vi "Channel Selection Dialog.vi"(7 "DisplayFilter":u8(ring)=7 items=["K_CHAN_R", "K_CHAN_W", "K_CHAN_RW", "K_CHAN_VOLT", "K_CHAN_FAULT", "K_ALL", "K_CUSTOM", "K_CHAN_R_VIS", "K_CHAN_W_VIS", "K_CHAN_RW_VIS", "K_CHAN_VOLT_VIS", "K_CHAN_FAULT_VIS"], 8 "error in (no error)":errorcluster, 9 "NIVS.System Definition Root":refnum<k24>, 10 "Start NodePath":string, 11 "Start NodePathArray":string[](array[string])) -> (0 "error out":errorcluster, 1 "Cancelled?":bool, 2 "Selected NodePath":string, 3 "Selected NodePathArray":string[](array[string]))   [LabVIEW 2011]
doc: "Use this template to create a dialog box with event handling."
uses:
  NationalInstruments.VeriStand.SystemStorageUI
  NationalInstruments.VeriStand.SystemStorage
  <vilib>/NI Veristand/UI Controls/Single Node Browser/NI_VS UI Single Node Browser.lvlib
panel:
  in  "Cancel":bool
  in  "Ok":bool
  in  "Selected Channel":refnum<k24>(container)
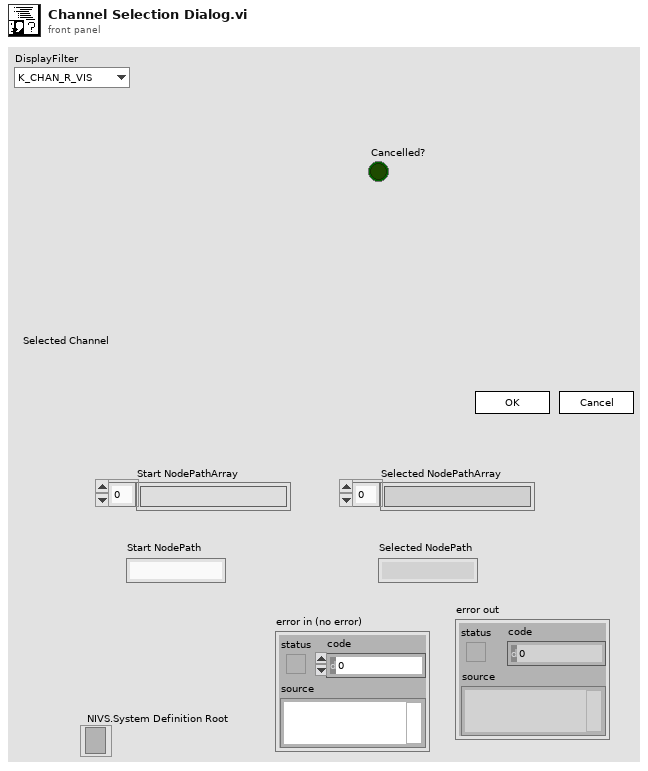
[diagram p1: front panel]
types:
  T1 = typedef "NI_VS UI Single Node Browser.lvlib/Callback Type.ctl" = cluster{"Net Callbacks":refnum<k27>[], "Event":refnum<user-event>}
  T2 = typedef "NI_VS UI Single Node Browser.lvlib/Node Ref.ctl" = refnum<k24>
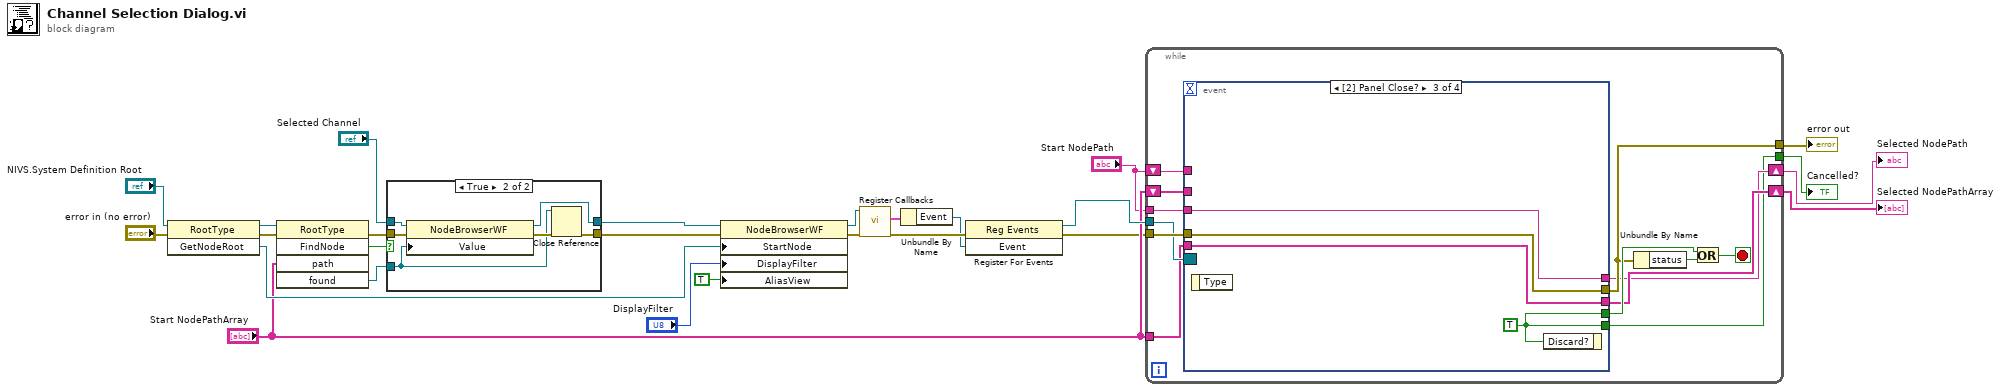
[diagram p0: block diagram]
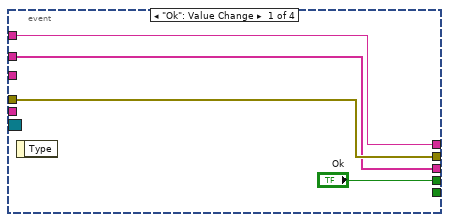
[diagram p3: hidden frame]
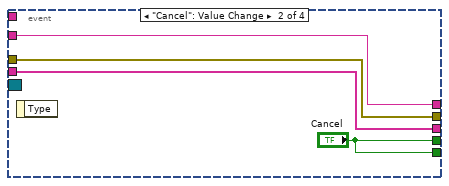
[diagram p4: hidden frame]
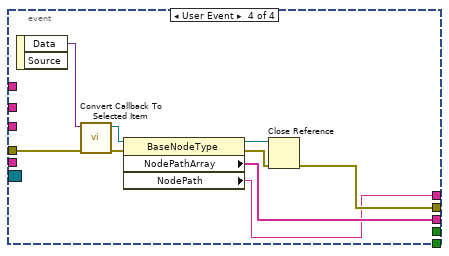
[diagram p5: hidden frame]
diagram:
  n1 = invoke class="RootType" method="GetNodeRoot"(reference="NIVS.System Definition Root", error in="error in (no error)") -> (reference out=w20:refnum<k24>, error out=w21:errorcluster, "GetNodeRoot"=w19:refnum<k24>)  [unwired: 1 in]
  n2 = invoke class="RootType" method="FindNode"(reference=w20, error in=w21, "path"="Start NodePathArray") -> (error out=w12:errorcluster, "FindNode"=w10:bool, "found"=w13:refnum<k24>)  [unwired: 2 in, 2 out]
  n3 = case shown="True" w10 {
    tunnel: w13 -> [_ w29]
    tunnel: w12 -> [w28 w30]
    tunnel: [w28 w33] -> w11
    tunnel: "Selected Channel" -> [w27 w32]
    tunnel: [w27 w31] -> w9
    frame False {
    }
    frame True {
      n4 = property class="NodeBrowserWF"(reference=w32, error in=w30, "Value"=w29) -> (reference out=w31:refnum<k24>, error out=w34:errorcluster)
      n5 = Close Reference(reference=w29, error in (no error)=w34) -> (error out=w33:errorcluster)
    }
  }
  n6 = property class="NodeBrowserWF"(reference=w9, error in=w11, "StartNode"=w19, "DisplayFilter"="DisplayFilter", "AliasView"=TRUE) -> (reference out=w16:refnum<k24>, error out=w17:errorcluster)
  n7 = call <vilib>:"Register Callbacks.vi"("error in (no error)"=w17, "Single Node Browser"=w16) -> ("error out"=w25:errorcluster, "Callbacks"=w18:T1)  [unwired: 7 in, 1 out]
  n8 = Unbundle By Name(w18) -> ("Event"=w8:refnum<user-event>)
  n9 = register-events(error in=w25, w8) -> (reference out=w24:refnum<event-registration>, error out=w1:errorcluster)  [unwired: 1 in]
  n10 = while {
    tunnel: [w45] -> w26
    tunnel: w1 -> [w46]
    tunnel: w24 -> [w42]
    shift-right: [w41] -> w7
    shift-left: "Start NodePathArray" -> [w40]
    tunnel: "Start NodePathArray" -> [w39]
    shift-right: [w38] -> w5
    shift-left: "Start NodePath" -> [w37]
    tunnel: "Start NodePath" -> [w36]
    tunnel: [w35] -> w3
    stop <- w44 stop-if-true
    n11 = event shown="[2] Panel Close?" {
      selector: w42 -> [_ _ _ _]
      dyn-events: _ -> [_ _ _ _]
      timeout: _ -> [_ _ _ _]
      tunnel: ["Ok" "Cancel" w56 _] -> w47
      tunnel: [w51 w55 w59 w66] -> w45
      tunnel: w46 -> [w51 w55 w59 w67]
      tunnel: [w49 w54 w58 w61] -> w41
      tunnel: w40 -> [w49 _ _ _]
      tunnel: w39 -> [_ w54 w58 _]
      tunnel: [w48 w53 w57 w60] -> w38
      tunnel: w37 -> [w48 _ _ _]
      tunnel: w36 -> [_ w53 w57 _]
      tunnel: [_ "Cancel" w56 _] -> w35
      event "Ok": Value Change {
        n12 = event-data() -> ()  [unwired: 1 in, 1 out]
      }
      event "Cancel": Value Change {
        n13 = event-data() -> ()  [unwired: 1 in, 1 out]
      }
      event Panel Close? {
        w56 = TRUE ("Cancel")
        n14 = event-data() -> ()  [unwired: 1 in, 1 out]
        n15 = event-data("Discard?"=w56) -> ()  [unwired: 1 in, 1 out]
      }
      event User Event {
        n16 = event-data() -> ("Data"=w68:variant)  [unwired: 1 in, 1 out]
        n17 = call <vilib>:"Convert Callback To Selected Item.vi"("error in"=w67, "Data"=w68) -> ("error out"=w62:errorcluster, "Selected Item"=w65:T2)  [unwired: 8 in]
        n18 = property class="BaseNodeType"(reference=w65, error in=w62) -> (reference out=w64:T2, error out=w63:errorcluster, "NodePathArray"=w61:string[], "NodePath"=w60:string)
        n19 = Close Reference(reference=w64, error in (no error)=w63) -> (error out=w66:errorcluster)
      }
    }
    n20 = Unbundle By Name(w45) -> ("status"=w43:bool)
    n21 = Or(x=w47, y=w43) -> (x .or. y?=w44:bool)
  }
  "error out" <- w26
  "Selected NodePathArray" <- w7
  "Selected NodePath" <- w5
  "Cancelled?" <- w3
